vi "ConvertStringToFloat_Array-1D.vi"(7 "default value (NaN)":dbl=nan format="%#_13g", 11 "String":string[](array[string])) -> (3 "Array of Doubles":dbl[](array[numeric]), 5 "error out":errorcluster)   [LabVIEW 2022 SP3, in "hse-misc.lvlib"]
doc: "converts array of string values to floating point values\n\n____\nHAMPEL SOFTWARE ENGINEERING v3.8.0 (2023-12-18 14:41)"
uses:
  hse-misc.lvlib
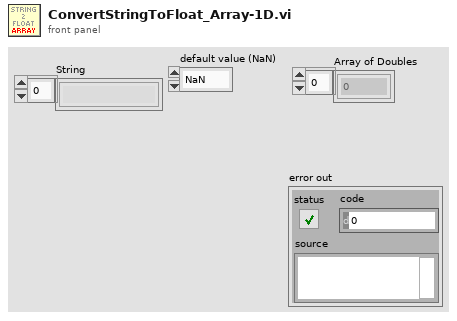
[diagram p1: front panel]
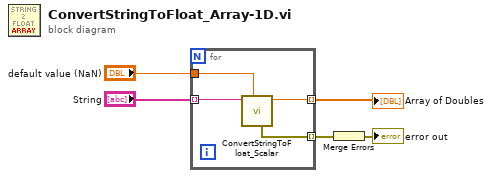
[diagram p0: block diagram]
diagram:
  n1 = for {
    tunnel: "String" -> [w9] mode=indexing
    tunnel: [w8] -> w4 mode=indexing
    tunnel: [w7] -> w3 mode=indexing
    tunnel: "default value (NaN)" -> [w6]
    n2 = call "ConvertStringToFloat_Scalar.vi"("default value (NaN)"=w6, "String"=w9) -> ("Double"=w8:dbl, "error out"=w7:errorcluster)  [unwired: 8 in]
  }
  "Array of Doubles" <- w4
  n3 = Merge Errors(w3) -> (→"error out":errorcluster)
